vi "Sort Signals By Frame Order.vi"(8 "error in (no error)":errorcluster, 9 "Node Refs":i32[](array[numeric]), 10 "XNET Paths":string[](array[string]), 11 "Signals":T1[](array[typedef]) {"Data Type" items=["Signed", "Unsigned", "IEEE Float"]}) -> (0 "error out":errorcluster, 1 "Ordered Node Refs":i32[](array[numeric]), 2 "Ordered XNET Paths":string[](array[string]), 3 "Ordered Signals":T1[](array[typedef]) {"Data Type" items=["Signed", "Unsigned", "IEEE Float"]})   [LabVIEW 2019, in "Protection and Counter Support System Explorer.lvlib"]
uses:
  Protection and Counter Support System Explorer.lvlib
  <vilib>/xnet/xnet.llb/XNET Create Session (Conversion).vi
  <vilib>/xnet/xnet.llb/XNET Convert (Signal to Frame CAN).vi
  Shared/Types/XNET Signal Configuration.ctl
  Shared/Protection and Counter Support Shared.lvlib
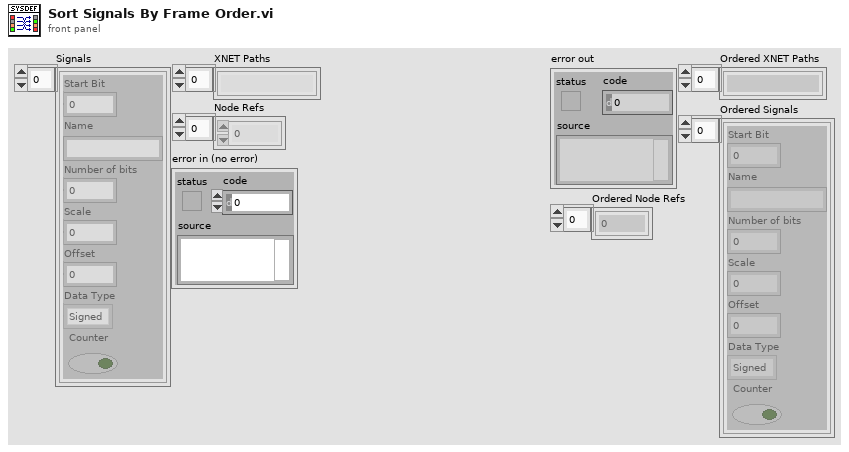
[diagram p1: front panel]
types:
  T1 = typedef "Protection and Counter Support Shared.lvlib/XNET Signal Configuration.ctl" = cluster{"Start Bit":i32, "Name":string, "Number of bits":i32, "Scale":dbl, "Offset":dbl, "Data Type":u32, "Counter":bool}
  T2 = typedef "XNET Frame CAN.ctl" = cluster{"timestamp":timestamp, "payload":u8[], "identifier":u32, "type":T3, "extended?":bool, "echo?":bool}
  T3 = typedef "XNET Frame Type CAN.ctl" = u8
  T4 = cluster{"index of element":i32, string, "MonitoredChannelSettings":T1, "index of element":i32}
  T5 = cluster{"index of element":i32, string, "MonitoredChannelSettings":T1, "index of element":i32}[]
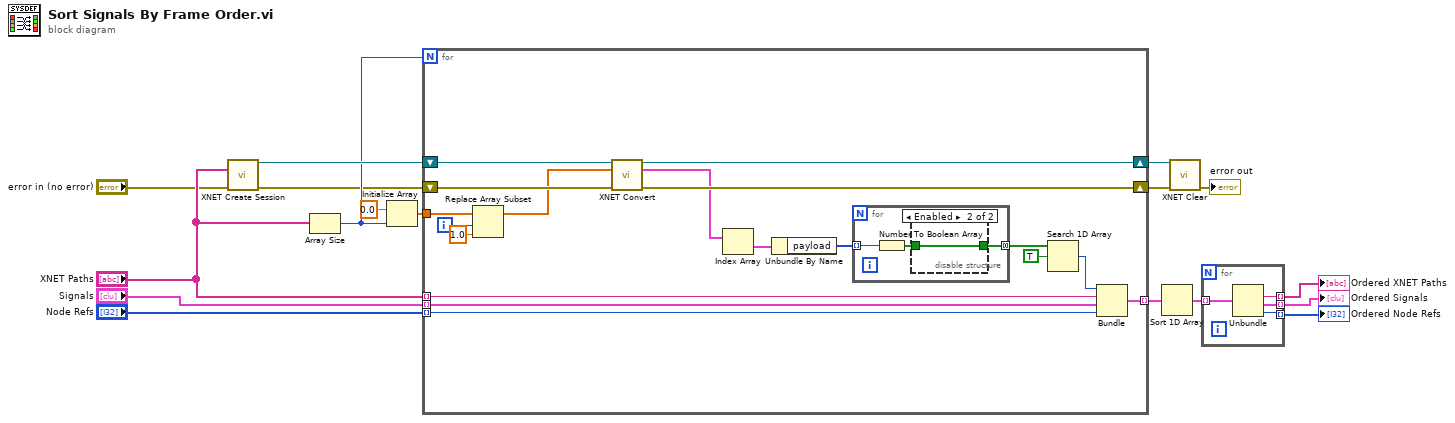
[diagram p0: block diagram]
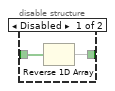
[diagram p2: hidden frame]
diagram:
  n1 = call-poly <vilib>:"XNET Create Session.vi"("signal list"="XNET Paths", "error in (no error)"="error in (no error)") -> ("session out"=w17:refnum<k21>, "error out"=w13:errorcluster)  [unwired: 12 in]
  n2 = Array Size(array="XNET Paths") -> (size(s)=w14:i32)
  n3 = Initialize Array(0.0 ("element"), w14) -> (w15:dbl[])
  n4 = for {
    N: w14 -> [_]
    tunnel: w15 -> [w34]
    shift-right: [w30] -> w7
    shift-left: w13 -> [w31]
    tunnel: "XNET Paths" -> [w27] mode=indexing
    tunnel: [w26] -> w12 mode=indexing
    tunnel: "Signals" -> [w20] mode=indexing
    tunnel: "Node Refs" -> [w19] mode=indexing
    shift-right: [w18] -> w6
    shift-left: w17 -> [w35]
    i -> [w33]
    n5 = Replace Array Subset(array=w34, new element=1.0 ("new element/subarray"), index=w33) -> (w21:dbl[])
    n6 = call-poly <vilib>:"XNET Convert.vi"("session in"=w35, "signal data"=w21, "error in (no error)"=w31) -> ("session out"=w18:refnum<k21>, "frame data"=w29:T2[], "error out"=w30:errorcluster)  [unwired: 9 in, 1 out]
    n7 = Index Array(array=w29) -> (element=w28:T2)  [unwired: 1 in]
    n8 = Unbundle By Name(w28) -> ("payload"=w25:u8[])
    n9 = for {
      tunnel: w25 -> [w38] mode=indexing
      tunnel: [w36] -> w24 mode=concatenating
      n10 = Number To Boolean Array(number=w38) -> (Boolean array=w37:bool[])
      n11 = disable-structure shown="Enabled" {
        disable-tunnel: w37 -> [w40 w41]
        disable-tunnel: [w39 w41] -> w36
        frame Disabled {
          n12 = Reverse 1D Array(array=w40) -> (reversed array=w39:bool[])
        }
        frame Enabled {
        }
      }
    }
    n13 = Search 1D Array(1D array=w24, element=TRUE) -> (index of element=w22:i32)  [unwired: 1 in]
    n14 = Bundle("index of element"=w22, w27, "MonitoredChannelSettings"=w20, "index of element"=w19) -> (w26:T4)  [unwired: 1 in]
  }
  n15 = Sort 1D Array(array=w12) -> (sorted array=w1:T5)
  n16 = call <vilib>:"XNET Clear.vi"("session in"=w6, "error in (no error)"=w7) -> ("error out"=→"error out":errorcluster)  [unwired: 13 in]
  n17 = for {
    tunnel: w1 -> [w45] mode=indexing
    tunnel: [w44] -> w4 mode=indexing
    tunnel: [w43] -> w3 mode=indexing
    tunnel: [w42] -> w2 mode=indexing
    n18 = Unbundle(w45) -> (w44:string, "MonitoredChannelSettings"=w43:T1, "index of element"=w42:i32)  [unwired: 1 out]
  }
  "Ordered XNET Paths" <- w4
  "Ordered Signals" <- w3
  "Ordered Node Refs" <- w2
